vi "PID-Parameter Druckregler.vi"() -> ()   [LabVIEW 2020, in "Erweiterte Konfig.lvlib"]
uses:
  Erweiterte Konfig.lvlib
  Visualisierungs Elemente/Zahlen-Eingabefeld.ctl
  cRIO/PC/Kommunikation mit cRIO.lvlib
  cRIO/PC/Aktionen FGV Druckregler.ctl
panel:
  in  "FT-IR Regler -":T1 format="%#_5g"
  in  "FT-IR Regler +":T1 format="%#_5g"
  in  "FT-IR OUT -":T1 format="%#_5g"
  in  "FT-IR OUT +":T1 format="%#_5g"
  in  "FT-IR D":T1 format="%#_5g"
  in  "FT-IR I":T1 format="%#_5g"
  in  "FT-IR P":T1 format="%#_5g"
  in  "FT-IR Regler Toleranz":bool
  in  "FT-IR OUT Toleranz":bool
  in  "Filter Regler -":T1 format="%#_5g"
  in  "Filter Regler +":T1 format="%#_5g"
  in  "Filter OUT -":T1 format="%#_5g"
  in  "Filter OUT +":T1 format="%#_5g"
  in  "Filter D":T1 format="%#_5g"
  in  "Filter I":T1 format="%#_5g"
  in  "Filter P":T1 format="%#_5g"
  in  "Filter Regler Toleranz":bool
  in  "Filter OUT Toleranz":bool
  in  "BEENDEN":bool
  # "PID Parameter Druck-Regler"
  # "Druck Filterkammer"
  # "Durchfluss FT-IR"
  # "Verstärkung KR:"
  # "Verstärkung KR:"
  # "Nachstellzeit TN:"
  # "Nachstellzeit TN:"
  # "sec"
  # "sec"
  # "Vorhaltezeit TD:"
  # "Vorhaltezeit TD:"
  # "sec"
  # "sec"
  # "OUT Toleranz +:"
  # "%"
  # "OUT Toleranz +:"
  # "%"
  # "OUT Toleranz -:"
  # "OUT Toleranz -:"
  # "%"
  # "%"
  # "mbar"
  # "l/min"
  # "Regler Toleranz +:"
  # "Regler Toleranz +:"
  # "Regler Toleranz -:"
  # "mbar"
  # "Regler Toleranz -:"
  # "l/min"
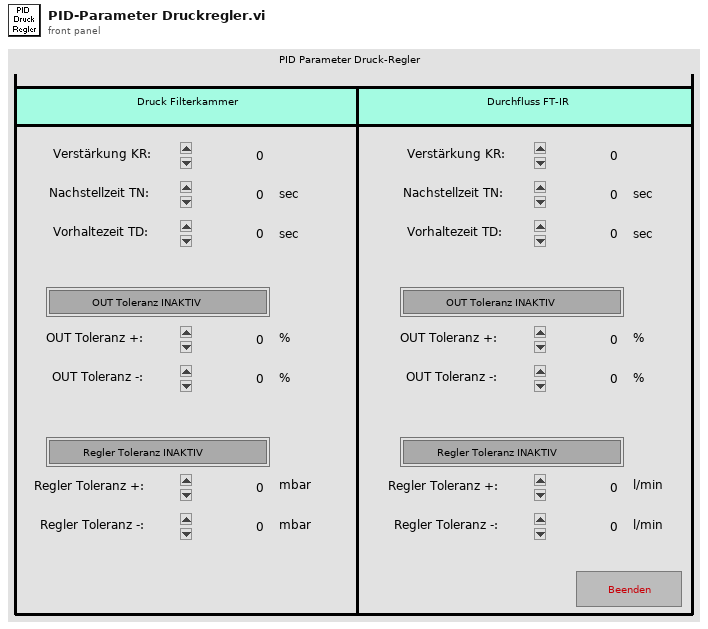
[diagram p1: front panel]
types:
  T1 = typedef "Zahlen-Eingabefeld.ctl" = sgl
  T2 = typedef "Kommunikation mit cRIO.lvlib/Aktionen FGV Druckregler.ctl" = enum16{"lesen", "Parameter", "Istwerte", "laden", "speichern"}
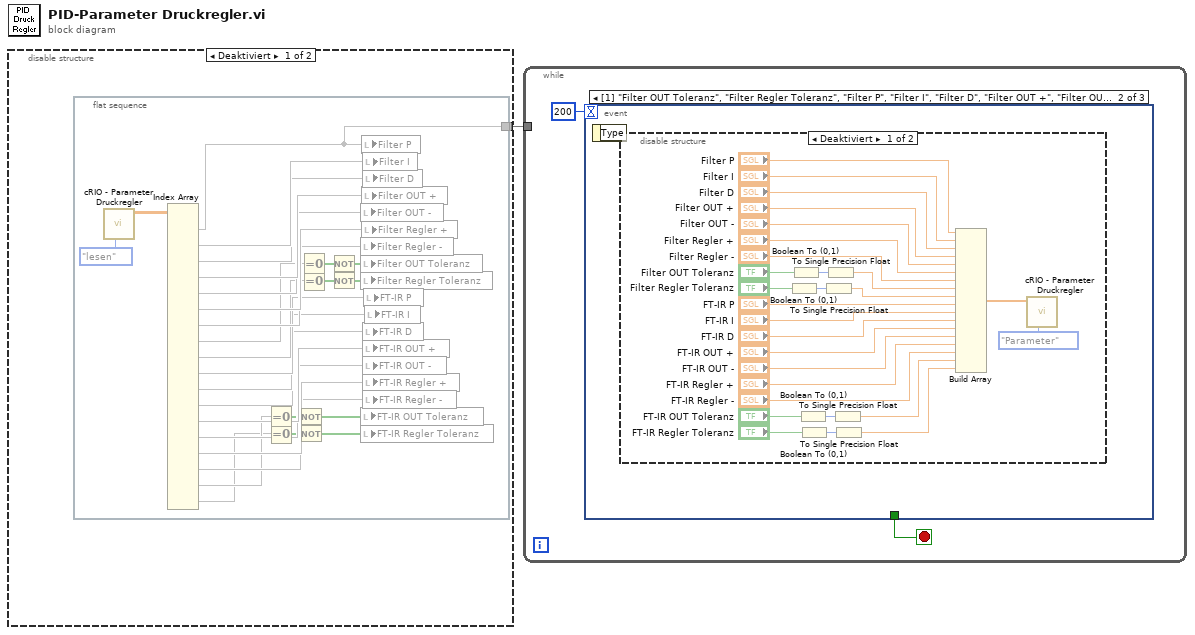
[diagram p0: block diagram]
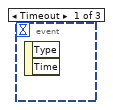
[diagram p3: hidden frame]
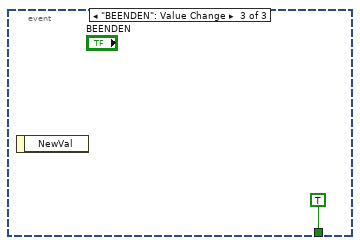
[diagram p5: hidden frame]
diagram:
  n1 = disable-structure shown="Deaktiviert" {
    disable-tunnel: [w2 _] -> w1
    frame Disabled {
      n2 = flat-sequence {
        tunnel: [w4] -> w2
        frame #0 {
          n3 = call "cRIO - Parameter Druckregler.vi"("Aktion"=Aktionen_FGV_Druckregler."lesen") -> ("Parameter Regler"=w30:sgl[][])  [unwired: 7 in, 3 out]
          n4 = Index Array(array=w30) -> (element #1=w4:sgl[], element #2=w29:sgl[], element #3=w28:sgl[], element #4=w27:sgl[], element #5=w26:sgl[], element #6=w25:sgl[], element #7=w24:sgl[], element #8=w23:sgl[], element #9=w22:sgl[], element #10=w17:sgl[], element #11=w16:sgl[], element #12=w15:sgl[], element #13=w14:sgl[], element #14=w13:sgl[], element #15=w12:sgl[], element #16=w11:sgl[], element #17=w6:sgl[], element #18=w5:sgl[])  [unwired: 36 in]
          n5 = Equal To 0?(x=w6) -> (x = 0?=w10:bool[])
          n6 = Equal To 0?(x=w5) -> (x = 0?=w9:bool[])
          n7 = Not(x=w10) -> (.not. x?=w8:bool[])
          n8 = Not(x=w9) -> (.not. x?=w7:bool[])
          n9 = Equal To 0?(x=w23) -> (x = 0?=w20:bool[])
          n10 = Equal To 0?(x=w22) -> (x = 0?=w21:bool[])
          n11 = Not(x=w20) -> (.not. x?=w19:bool[])
          n12 = Not(x=w21) -> (.not. x?=w18:bool[])
          n13 = local write "Filter OUT -"(w26) -> ()
          n14 = local write "Filter Regler -"(w24) -> ()
          n15 = local write "Filter OUT Toleranz"(w19) -> ()
          n16 = local write "Filter Regler Toleranz"(w18) -> ()
          n17 = local write "FT-IR OUT Toleranz"(w8) -> ()
          n18 = local write "FT-IR Regler Toleranz"(w7) -> ()
          n19 = local write "Filter P"(w4) -> ()
          n20 = local write "Filter OUT +"(w27) -> ()
          n21 = local write "Filter Regler +"(w25) -> ()
          n22 = local write "Filter I"(w29) -> ()
          n23 = local write "Filter D"(w28) -> ()
          n24 = local write "FT-IR D"(w15) -> ()
          n25 = local write "FT-IR OUT +"(w14) -> ()
          n26 = local write "FT-IR OUT -"(w13) -> ()
          n27 = local write "FT-IR Regler +"(w12) -> ()
          n28 = local write "FT-IR Regler -"(w11) -> ()
          n29 = local write "FT-IR P"(w17) -> ()
          n30 = local write "FT-IR I"(w16) -> ()
        }
      }
    }
    frame Enabled {
    }
  }
  n31 = while {
    tunnel: w1 -> [_]
    stop <- w32 stop-if-true
    n32 = event shown="[1] \"Filter OUT Toleranz\", \"Filter Regler Toleranz\", \"Filter P\", \"Filter I\", \"Filter D\", \"Filter OUT +\", \"Filter OUT -\", \"Filter Regler +\", \"Filter Regler -\", \"FT-IR OUT Toleranz\", \"FT-IR Regler Toleranz\", \"FT-IR P\", \"FT-IR I\", \"FT-IR D\", \"FT-IR OUT +\", \"FT-IR OUT -\", \"FT-IR Regler +\", \"FT-IR Regler -\": Wertänderung" {
      selector: _ -> [_ _ _]
      dyn-events: _ -> [_ _ _]
      timeout: 200 -> [_ _ _]
      tunnel: [_ _ TRUE ("ABBRECHEN")] -> w32
      event Timeout {
        n33 = event-data() -> ()  [unwired: 1 in, 2 out]
      }
      event "Filter OUT Toleranz", "Filter Regler Toleranz", "FT-IR OUT Toleranz", "FT-IR Regler Toleranz": Value Change {
        n34 = event-data() -> ()  [unwired: 1 in, 1 out]
        n35 = disable-structure shown="Deaktiviert" {
          frame Disabled {
            n36 = Boolean To (0,1)(Boolean="Filter Regler Toleranz") -> (0, 1=w58:i16)
            n37 = Boolean To (0,1)(Boolean="Filter OUT Toleranz") -> (0, 1=w59:i16)
            n38 = Boolean To (0,1)(Boolean="FT-IR OUT Toleranz") -> (0, 1=w57:i16)
            n39 = Boolean To (0,1)(Boolean="FT-IR Regler Toleranz") -> (0, 1=w56:i16)
            n40 = To Single Precision Float(number=w58) -> (single precision float=w44:sgl)
            n41 = To Single Precision Float(number=w59) -> (single precision float=w45:sgl)
            n42 = To Single Precision Float(number=w57) -> (single precision float=w36:sgl)
            n43 = To Single Precision Float(number=w56) -> (single precision float=w35:sgl)
            n44 = Build Array("Filter P", "Filter I", "Filter D", "Filter OUT +", "Filter OUT -", "Filter Regler +", "Filter Regler -", w45, w44, "FT-IR P", "FT-IR I", "FT-IR D", "FT-IR OUT +", "FT-IR OUT -", "FT-IR Regler +", "FT-IR Regler -", w36, w35) -> (w34:T1[])
            n45 = call "cRIO - Parameter Druckregler.vi"("Aktion"=Aktionen_FGV_Druckregler."Parameter", "Parameter Regler"=w34) -> ()  [unwired: 6 in, 4 out]
          }
          frame Enabled {
          }
        }
      }
      event "BEENDEN": Value Change {
        n46 = event-data() -> ()  [unwired: 1 in, 1 out]
      }
    }
  }
